vi "APPA109N - One measurement.vi"() -> ()   [LabVIEW 2016]
uses:
  <vilib>/Instr/_visa.llb/VISA Configure Serial Port (Instr).vi
panel:
  out "Number (sub-panel)":dbl
  out "Checksum":bool
  out "Units":T1(ring)
  out "Number":dbl
  out "Regime":string
  in  "Multimeter Port":refnum<visa-resource-name>="COM3"
  # "Press button while turning meter on from OFF position.\nRANGE : Turn off beeper.\nBLUE : Disable Auto Power OFF."
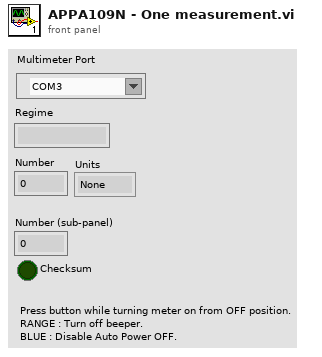
[diagram p1: front panel]
types:
  T1 = enum16{"None", "V", "mV", "A", "mA", "dB", "dBm", "nF", "uF", "mF", "Ohm", "kOhm", "MOhm", "GOhm", "%", "Hz", "kHz", "MHz", "C", "F", "s", "ms", "ns", "V (manual)", "mV (manual)", "A (manual)", "mA (manual)", "Ohm (manual)", "kOhm (maual)", "MOhm (manual)", ""}
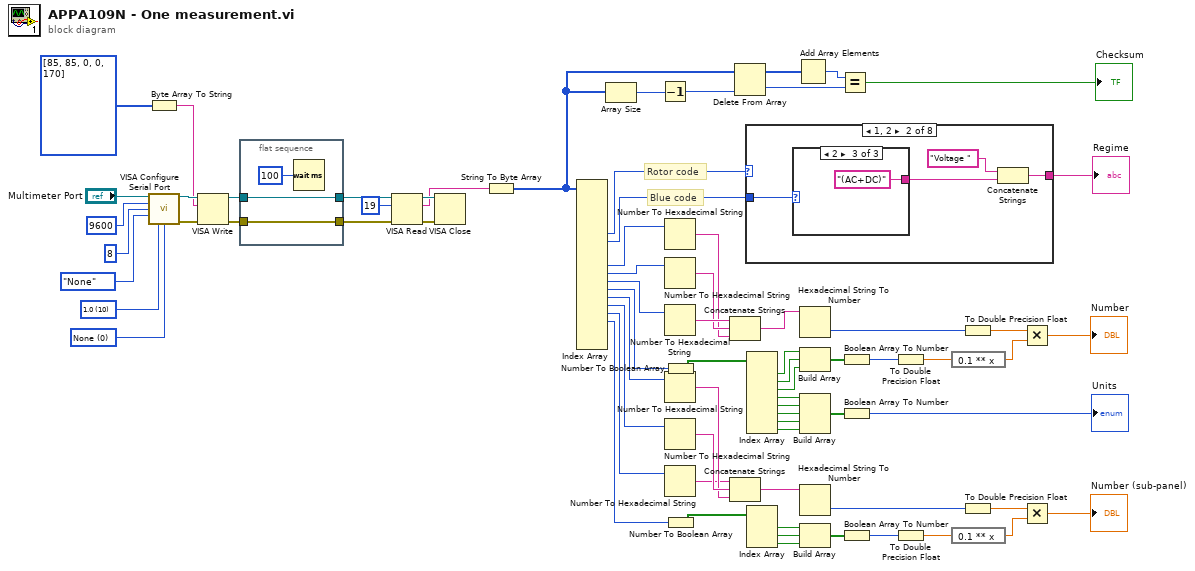
[diagram p0: block diagram]
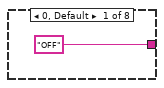
[diagram p2: hidden frame]
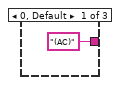
[diagram p3: hidden frame]
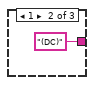
[diagram p4: hidden frame]
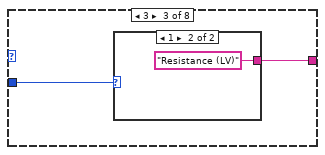
[diagram p5: hidden frame]
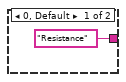
[diagram p6: hidden frame]
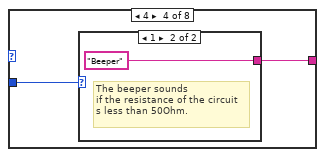
[diagram p7: hidden frame]
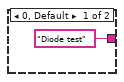
[diagram p8: hidden frame]
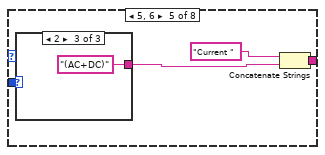
[diagram p9: hidden frame]
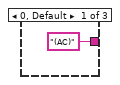
[diagram p10: hidden frame]
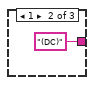
[diagram p11: hidden frame]
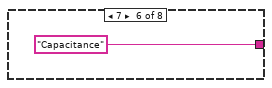
[diagram p12: hidden frame]
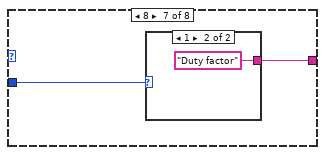
[diagram p13: hidden frame]
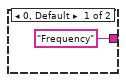
[diagram p14: hidden frame]
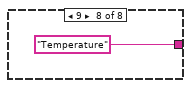
[diagram p15: hidden frame]
diagram:
  w68 = u16 0 items=["None", "XON/XOFF", "RTS/CTS", "XON/XOFF & RTS/CTS", "DTR/DSR", "XON/XOFF & DTR/DSR"] ("flow control (0:none)")
  w69 = u16 10 items=["1.0"=10, "1.5"=15, "2.0"=20] ("stop bits (10: 1 bit)")
  # "Blue code"
  # "Rotor code"
  n1 = Byte Array To String(unsigned byte array=i32[] [85, 85, 0, 0, 170]) -> (string=w57:string)
  n2 = call-poly "VISA Configure Serial Port"("VISA resource name"="Multimeter Port", "baud rate (9600)"=u32 9600, "data bits (8)"=u16 8, "parity (0:none)"=enum16{"None", "Odd", "Even", "Mark", "Space"}."None", "stop bits (10: 1 bit)"=w69, "flow control (0:none)"=w68) -> ("VISA resource name out"=w65:refnum<visa-resource-name>, "error out"=w64:errorcluster)  [unwired: 8 in]
  n3 = VISA Write(VISA resource name=w65, write buffer=w57, error in (no error)=w64) -> (VISA resource name out=w67:refnum<visa-resource-name>, error out=w66:errorcluster)  [unwired: 1 out]
  n4 = flat-sequence {
    tunnel: w67 -> [w75]
    tunnel: w66 -> [w74]
    tunnel: [w75] -> w63
    tunnel: [w74] -> w62
    frame #0 {
      n5 = Wait (ms)(milliseconds to wait=u32 100) -> ()  [unwired: 1 out]
    }
  }
  n6 = VISA Read(VISA resource name=w63, byte count=u32 19, error in (no error)=w62) -> (VISA resource name out=w61:refnum<visa-resource-name>, read buffer=w56:string, error out=w60:errorcluster)  [unwired: 1 out]
  n7 = VISA Close(VISA resource name=w61, error in (no error)=w60) -> ()  [unwired: 1 out]
  n8 = String To Byte Array(string=w56) -> (unsigned byte array=w28:u8[])
  n9 = Index Array(array=w28) -> (element #5=w55:u8, element #6=w54:u8, element #9=w51:u8, element #10=w52:u8, element #11=w53:u8, element #12=w46:u8, element #13=w17:u8, element #14=w16:u8, element #15=w15:u8, element #16=w6:u8)  [unwired: 19 in, 9 out]
  n10 = Array Size(array=w28) -> (size(s)=w29:i32)
  n11 = Decrement(x=w29) -> (x-1=w27:i32)
  n12 = Number To Hexadecimal String(2:w51) -> (0:w48:string)  [unwired: 1 in]
  n13 = Number To Hexadecimal String(2:w52) -> (0:w49:string)  [unwired: 1 in]
  n14 = Number To Hexadecimal String(2:w53) -> (0:w50:string)  [unwired: 1 in]
  n15 = Number To Hexadecimal String(2:w17) -> (0:w22:string)  [unwired: 1 in]
  n16 = Number To Hexadecimal String(2:w16) -> (0:w23:string)  [unwired: 1 in]
  n17 = Number To Hexadecimal String(2:w15) -> (0:w18:string)  [unwired: 1 in]
  n18 = Number To Boolean Array(number=w46) -> (Boolean array=w45:bool[])
  n19 = Number To Boolean Array(number=w6) -> (Boolean array=w14:bool[])
  n20 = Concatenate Strings(w50, w49, w48) -> (w47:string)
  n21 = Concatenate Strings(w18, w23, w22) -> (w21:string)
  n22 = Delete From Array(array=w28, index=w27) -> (deleted portion=w24:u8, array with subset deleted=w26:u8[])  [unwired: 1 in]
  n23 = case shown="1, 2" w55 {
    tunnel: ["OFF" w79 w86 w89 w93 "Capacitance" w101 "Temperature"] -> w3
    tunnel: w54 -> [_ w81 w85 w90 w95 _ w102 _]
    frame 0, Default {
    }
    frame 1, 2 {
      n24 = case shown="2" w81 {
        tunnel: ["(AC)" "(DC)" "(AC+DC)"] -> w78
        frame 0, Default {
        }
        frame 1 {
        }
        frame 2 {
        }
      }
      n25 = Concatenate Strings("Voltage ", w78) -> (w79:string)
    }
    frame 3 {
      n26 = case shown="1" w85 {
        tunnel: ["Resistance" "Resistance (LV)"] -> w86
        frame 0, Default {
        }
        frame 1 {
        }
      }
    }
    frame 4 {
      n27 = case shown="1" w90 {
        tunnel: ["Diode test" "Beeper"] -> w89
        frame 0, Default {
        }
        frame 1 {
          # "The beeper sounds\nif the resistance of the circuit\ns less than 50Ohm."
        }
      }
    }
    frame 5, 6 {
      n28 = case shown="2" w95 {
        tunnel: ["(AC)" "(DC)" "(AC+DC)"] -> w96
        frame 0, Default {
        }
        frame 1 {
        }
        frame 2 {
        }
      }
      n29 = Concatenate Strings("Current ", w96) -> (w93:string)
    }
    frame 7 {
    }
    frame 8 {
      n30 = case shown="1" w102 {
        tunnel: ["Frequency" "Duty factor"] -> w101
        frame 0, Default {
        }
        frame 1 {
        }
      }
    }
    frame 9 {
    }
  }
  "Regime" <- w3
  n31 = Index Array(array=w45) -> (element #1=w44:bool, element #2=w43:bool, element #3=w42:bool, element #4=w35:bool, element #5=w34:bool, element #6=w33:bool, element #7=w32:bool, element #8=w31:bool)  [unwired: 8 in]
  n32 = Index Array(array=w14) -> (element #1=w13:bool, element #2=w12:bool, element #3=w11:bool)  [unwired: 3 in]
  n33 = Add Array Elements(numeric array=w26) -> (sum=w25:u8)
  n34 = Hexadecimal String To Number(string=w47) -> (number=w39:u32)  [unwired: 2 in, 1 out]
  n35 = Build Array(w44, w43, w42) -> (w41:bool[])
  n36 = Build Array(w35, w34, w33, w32, w31) -> (w30:bool[])
  n37 = Hexadecimal String To Number(string=w21) -> (number=w20:u32)  [unwired: 2 in, 1 out]
  n38 = Build Array(w13, w12, w11) -> (w10:bool[])
  n39 = Equal?(x=w25, y=w24) -> (x = y?=→"Checksum":bool)
  n40 = Boolean Array To Number(Boolean array=w41) -> (number=w40:u32)
  n41 = Boolean Array To Number(Boolean array=w30) -> (number=→"Units":u32)
  n42 = Boolean Array To Number(Boolean array=w10) -> (number=w9:u32)
  n43 = To Double Precision Float(number=w40) -> (double precision float=w37:dbl)
  n44 = To Double Precision Float(number=w9) -> (double precision float=w8:dbl)
  n45 = expression code="0.1 ** x"(w37) -> (w36:dbl)
  n46 = expression code="0.1 ** x"(w8) -> (w7:dbl)
  n47 = To Double Precision Float(number=w39) -> (double precision float=w38:dbl)
  n48 = To Double Precision Float(number=w20) -> (double precision float=w19:dbl)
  n49 = Multiply(x=w38, y=w36) -> (x*y=→"Number":dbl)
  n50 = Multiply(x=w19, y=w7) -> (x*y=→"Number (sub-panel)":dbl)
